vi "SLSC Switch Probe.vi"(11 "SLSC Switch out":refnum<class "SLSC Switch.lvclass">) -> (2 "Value String":string, 3 "Boolean":bool)   [LabVIEW 2015, in "SLSC Switch.lvclass"]
uses:
  Classes/SLSC Switch/SLSC Switch.lvclass
  Classes/SLSC Switch/Controls/Topology.ctl
  Classes/SLSC Switch/SLSC Switch.lvclass/SLSC Switch.ctl
panel:
  out "Topologies":T1[](array[typedef])
  out "Switch File Info":path
  out "session":refnum<k21>
  out "device":refnum<k21>
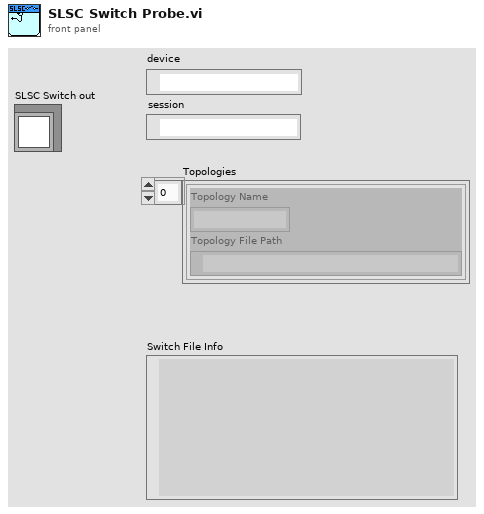
[diagram p1: front panel]
types:
  T1 = typedef "SLSC Switch.lvclass/Topology.ctl" = cluster{"Topology Name":string, "Topology File Path":path}
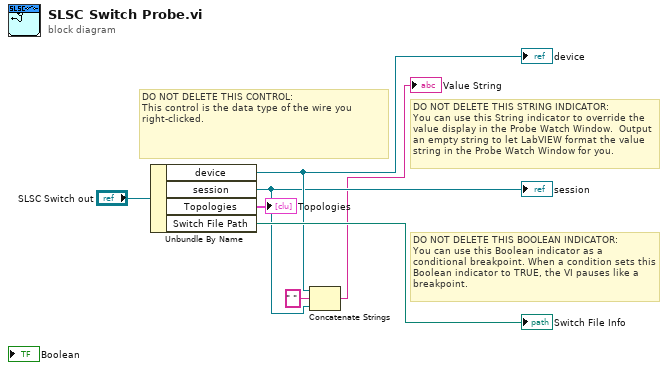
[diagram p0: block diagram]
diagram:
  # "DO NOT DELETE THIS STRING INDICATOR: \nYou can use this String indicator to override the value display in the Probe Watch Window.  Output an empty string to let LabVIEW format the value string in the Probe Watch Window for you."
  # "DO NOT DELETE THIS BOOLEAN INDICATOR: \nYou can use this Boolean indicator as a conditional breakpoint. When a condition sets this Boolean indicator to TRUE, the VI pauses like a breakpoint."
  # "DO NOT DELETE THIS CONTROL: \nThis control is the data type of the wire you right-clicked."
  n1 = Unbundle By Name("SLSC Switch out") -> ("device"=w5:refnum<k21>, "session"=w3:refnum<k21>, "Topologies"=→"Topologies":T1[], "Switch File Path"=→"Switch File Info":path)
  "device" <- w5
  "session" <- w3
  n2 = Concatenate Strings(w5, " " ("string"), w3) -> (→"Value String":string)
